vi "Verify CLI Echo Hello World.vi"(8 "error in":errorcluster) -> (0 "error out":errorcluster)   [LabVIEW 2020, in "Caraya Extension Tests.lvclass"]
uses:
  Caraya Extension Tests.lvclass
  Caraya Extension Tests.lvclass/Caraya Extension Tests.ctl
  <vilib>/addons/_JKI Toolkits/Caraya/classes/Test/Test.lvclass
  Source/Extensions/Caraya.Extension/Caraya.Extension.lvlib
  Source/Approval Tests/Approval Tests.lvlib
  Source/Approval Tests/OS Strings.ctl
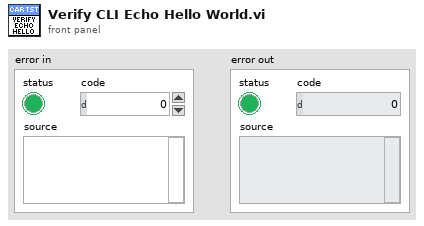
[diagram p1: front panel]
types:
  T1 = typedef "Approval Tests.lvlib/OS Strings.ctl" = cluster{"Windows":string, "Linux":string, "Mac":string}
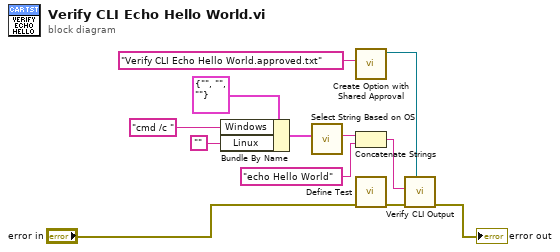
[diagram p0: block diagram]
diagram:
  n1 = Bundle By Name(cluster=T1 {"Windows"="", "Linux"="", "Mac"=""} ("Strings"), "Windows"="cmd /c ", "Linux"="") -> (w4:T1)
  n2 = call "Select String Based on OS.vi"("Strings"=w4) -> ("Selection"=w1:string)  [unwired: 10 in]
  n3 = call "Create Option with Shared Approval.vi"("Filename"="Verify CLI Echo Hello World.approved.txt") -> ("Options outs"=w6:refnum<class "Options.lvclass">)  [unwired: 10 in]
  n4 = Concatenate Strings(w1, "echo Hello World" ("command line")) -> (w8:string)
  n5 = call <vilib>:"Define Test.vi"("error in (no error)"="error in") -> ("error out"=w10:errorcluster)  [unwired: 9 in, 1 out]
  n6 = call "Verify CLI Output.vi"("Options"=w6, "error in"=w10, "command line"=w8) -> ("error out"=→"error out":errorcluster)  [unwired: 7 in, 1 out]
